vi "show CLFN calls.vi"() -> ()   [LabVIEW 2019]
uses:
  <vilib>/Utility/Data Type/Type Definitions/Data Type.ctl
  <vilib>/Utility/traverseref.llb/TRef TravTarget.ctl
  <vilib>/Utility/traverseref.llb/VI Scripting - Traverse.lvlib
  <vilib>/Utility/Data Type/NI_Data Type.lvlib
panel:
  out "Array":T1[](array[typedef])
  out "Array 2":string[](array[string])
  out "Calling Convention":u32
  out "Dynamic Library?":bool
  out "Parameter Info":T2(array[cluster])
  in  "search":string
  in  "file or folder":path
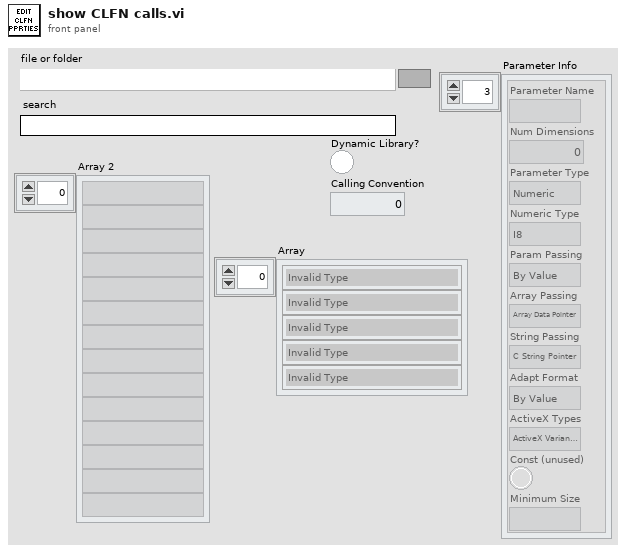
[diagram p1: front panel]
types:
  T1 = typedef "NI_Data Type.lvlib/Data Type.ctl" = enum8{"Invalid Type", "Void", "I8", "I16", "I32", "I64", "U8", "U16", "U32", "U64", "Single Float", "Double Float", "Extended Float", "Single Complex", "Double Complex", "Extended Complex", "Enum U8", "Enum U16", "Enum U32", "Enum U64", "Single Float With Unit", "Double Float With Unit", "Extended Float With Unit", "Single Complex with Unit", "Double Complex with Unit", "Extended Complex with Unit", "Boolean", "String", "Path", "Picture", "Tag", "Array", "Cluster", "Variant", "LV Variant", "Waveform", "Timestamp", "Digital Waveform", "Digital Data", "ExpressData", "Refnum", "External Data", "VI", "Poly VI", "LabVIEW Class Instance", "Fixed Point", "Set Collection", "Map Collection"}
  T2 = cluster{"Parameter Name":string, "Num Dimensions":i32, "Parameter Type":enum16{"Numeric", "Array", "String", "Waveform", "Digital Waveform", "Digital Table", "ActiveX", "Any", "Instance Data Pointer", "Void"}, "Numeric Type":enum16{"I8", "I16", "I32", "I64", "U8", "U16", "U32", "U64", "SGL", "DBL", "PTR INT", "PTR UINT"}, "Param Passing":enum16{"By Value", "Pointer To Value"}, "Array Passing":enum16{"Array Data Pointer", "Array Handle", "Array Handle Pointer"}, "String Passing":enum16{"C String Pointer", "Pascal String Pointer", "String Handle", "String Handle Pointer"}, "Adapt Format":enum16{"By Value", "Pointer To Value"}, "ActiveX Types":enum16{"ActiveX Variant Pointer", "IDispatch* Pointer", "IUnknown* Pointer"}, "Const (unused)":bool, "Minimum Size":string}[]
  T3 = typedef "TRef TravTarget.ctl" = enum16{"FP", "BD", "Other"}
  T4 = enum16{"I8", "I16", "I32", "I64", "U8", "U16", "U32", "U64", "SGL", "DBL", "PTR INT", "PTR UINT"}
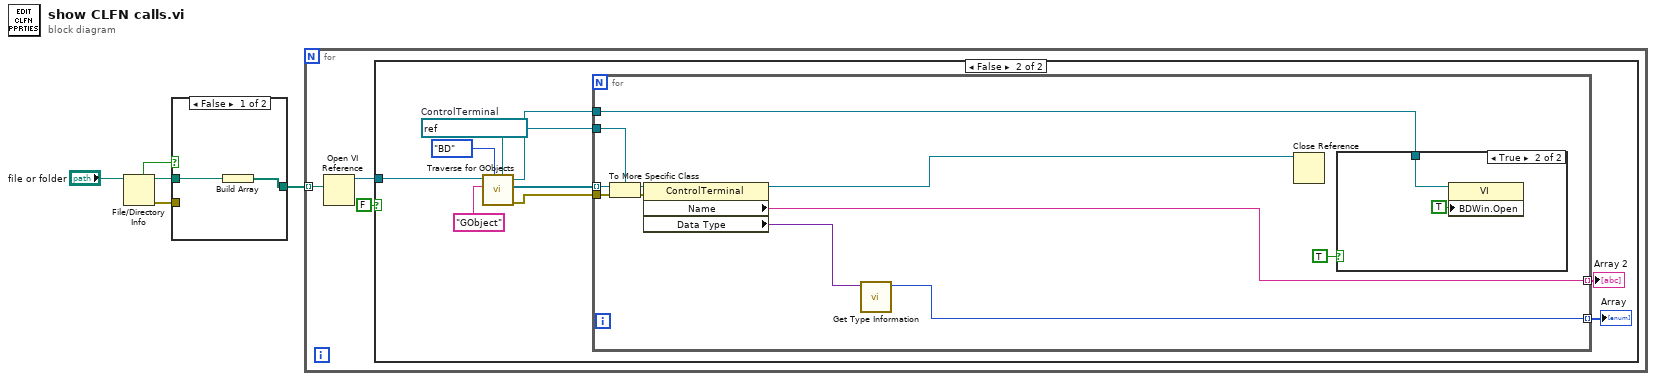
[diagram p0: block diagram]
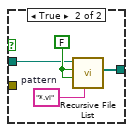
[diagram p2: hidden frame]
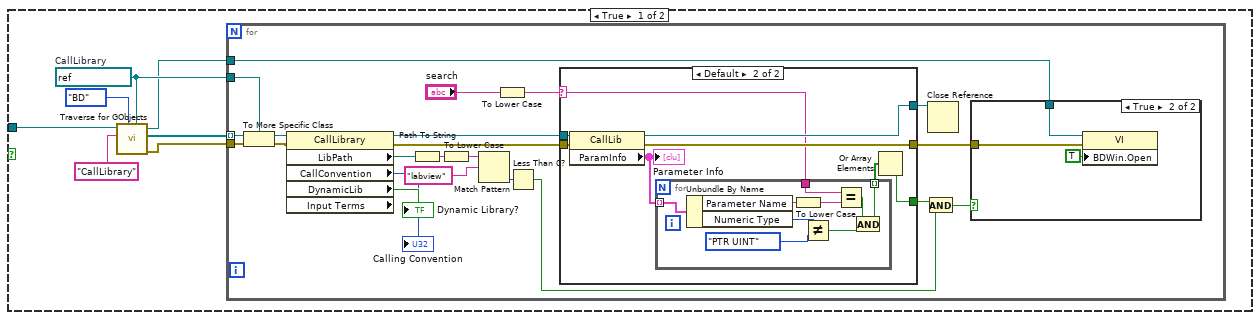
[diagram p3: hidden frame]
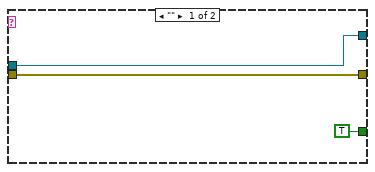
[diagram p4: hidden frame]
diagram:
  n1 = File/Directory Info(path="file or folder") -> (path out=w2:path, directory=w4:bool, error out=w1:errorcluster)  [unwired: 1 in, 4 out]
  n2 = case shown="False" w4 {
    tunnel: [w6 w9] -> w5
    tunnel: w2 -> [w7 w8]
    tunnel: w1 -> [_ _]
    frame False {
      n3 = Build Array(w7) -> (w6:path[])
    }
    frame True {
      w11 = FALSE
      w10 = "*.vi"  # pattern
      n4 = call <vilib>:"Recursive File List.vi"("pattern"=w10, "Continue Recursing on Error? (F)"=w11, "Treat LLBs as Folders?"=w11, "Folder Path"=w8) -> ("All Files in Dir"=w9:path[])  [unwired: 3 in, 4 out]
    }
  }
  n5 = for {
    tunnel: w5 -> [w13] mode=indexing
    n6 = Open VI Reference(vi path=w13) -> (vi reference=w14:refnum<vi>)  [unwired: 5 in, 1 out]
    n7 = case shown="False" FALSE {
      tunnel: w14 -> [w21 w75]
      frame True {
        w18 = refnum<vi> refnum  # CallLibrary
        n8 = call <vilib>:"Traverse for GObjects.vi"("Other Refnum"=w18, "Traverse Target"=TRef_TravTarget."BD", "Class Name"="CallLibrary", "VI Refnum"=w21) -> ("error out"=w17:errorcluster, "References"=w16:refnum<vi>[], "dup VI Refnum"=w15:refnum<vi>)  [unwired: 4 in, 1 out]
        n9 = for {
          tunnel: w16 -> [w43] mode=indexing
          tunnel: w18 -> [w42]
          tunnel: w17 -> [w41]
          tunnel: w15 -> [w33]
          n10 = To More Specific Class(target class=w42, reference=w43, error in=w41) -> (specific class reference=w40:refnum<vi>, error out=w39:errorcluster)
          n11 = property class="CallLibrary" props=["LibPath", "CallConvention", "DynamicLib", "Input Terms"](reference=w40, error in=w39) -> (reference out=w32:refnum<vi>, error out=w31:errorcluster, "LibPath"=w38:path, "CallConvention"=→"Calling Convention":u32, "DynamicLib"=→"Dynamic Library?":bool)  [unwired: 1 out]
          n12 = Path To String(path=w38) -> (string=w37:string)
          n13 = To Lower Case(string=w37) -> (all lower case string=w36:string)
          n14 = Match Pattern(string=w36, regular expression="labview") -> (offset past match=w34:i32)  [unwired: 1 in, 3 out]
          n15 = To Lower Case(string="search") -> (all lower case string=w24:string)
          n16 = Less Than 0?(x=w34) -> (x < 0?=w26:bool)
          n17 = case shown="Default" w24 {
            selector: w24 -> [_ w49]
            tunnel: w32 -> [w45 w54]
            tunnel: w31 -> [w46 w53]
            tunnel: [w46 w52] -> w30
            tunnel: [w45 w50] -> w28
            tunnel: [TRUE w47] -> w27
            frame "" {
            }
            frame Default {
              n18 = property class="CallLib"(reference=w54, error in=w53) -> (reference out=w50:refnum<vi>, error out=w52:errorcluster, "ParamInfo"=w51:T2)
              "Parameter Info" <- w51
              n19 = for {
                tunnel: w51 -> [w63] mode=indexing
                tunnel: w49 -> [w58]
                tunnel: [w57] -> w48 mode=indexing
                n20 = Unbundle By Name(w63) -> ("Parameter Name"=w59:string, "Numeric Type"=w62:T4)
                n21 = To Lower Case(string=w59) -> (all lower case string=w55:string)
                n22 = Not Equal?(x=w62, y=T4."PTR UINT" ("Numeric Type")) -> (x != y?=w60:bool)
                n23 = Equal?(x=w58, y=w55) -> (x = y?=w56:bool)
                n24 = And(x=w56, y=w60) -> (x .and. y?=w57:bool)
              }
              n25 = Or Array Elements(Boolean array=w48) -> (logical OR=w47:bool)
            }
          }
          n26 = And(x=w27, y=w26) -> (x .and. y?=w25:bool)
          n27 = Close Reference(reference=w28) -> ()  [unwired: 1 in, 1 out]
          n28 = case shown="True" w25 {
            tunnel: w30 -> [_ w64]
            tunnel: w33 -> [_ w65]
            frame False {
            }
            frame True {
              n29 = property class="VI"(reference=w65, error in=w64, "BDWin.Open"=TRUE ("Block Diagram Window:Open")) -> ()  [unwired: 2 out]
            }
          }
        }
      }
      frame False {
        w72 = refnum<vi> refnum  # ControlTerminal
        n30 = call <vilib>:"Traverse for GObjects.vi"("Other Refnum"=w72, "Traverse Target"=TRef_TravTarget."BD", "Class Name"="GObject", "VI Refnum"=w75) -> ("error out"=w71:errorcluster, "References"=w70:refnum<vi>[], "dup VI Refnum"=w69:refnum<vi>)  [unwired: 4 in, 1 out]
        n31 = for {
          tunnel: w70 -> [w86] mode=indexing
          tunnel: w72 -> [w85]
          tunnel: w71 -> [w84]
          tunnel: w69 -> [w81]
          tunnel: [w78] -> w68 mode=indexing
          tunnel: [w76] -> w67 mode=indexing
          n32 = To More Specific Class(target class=w85, reference=w86, error in=w84) -> (specific class reference=w83:refnum<vi>, error out=w82:errorcluster)
          n33 = property class="ControlTerminal"(reference=w83, error in=w82) -> (reference out=w80:refnum<vi>, "Name"=w78:string, "Data Type"=w77:variant)  [unwired: 1 out]
          n34 = call <vilib>:"Get Type Information.vi"("variant"=w77) -> ("type"=w76:T1)  [unwired: 6 in, 4 out]
          n35 = Close Reference(reference=w80) -> ()  [unwired: 1 in, 1 out]
          n36 = case shown="True" TRUE {
            tunnel: w81 -> [_ w87]
            frame False {
            }
            frame True {
              n37 = property class="VI"(reference=w87, "BDWin.Open"=TRUE ("Block Diagram Window:Open")) -> ()  [unwired: 1 in, 2 out]
            }
          }
        }
        "Array 2" <- w68
        "Array" <- w67
      }
    }
  }
